vi "getParametresEssai.vi"(8 "error in (no error)":errorcluster, 11 "VISA resource name":refnum<visa-resource-name>) -> (0 "error out":errorcluster, 2 "param out":T1, 3 "VISA resource name out":refnum<visa-resource-name>)   [LabVIEW 2023]
panel:
  out "read buffer":string
  out "Distance (mm)":dbl
  out "vitesse (mm/s)":dbl
  out "temps attente (ms)":i32
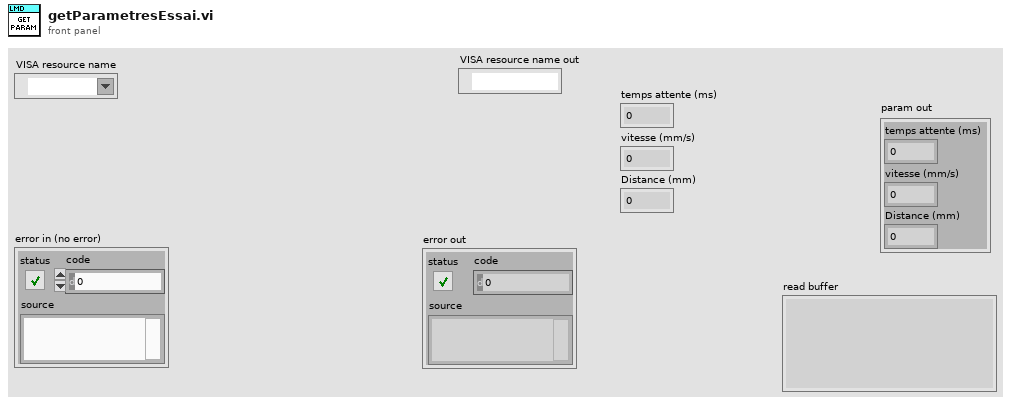
[diagram p1: front panel]
types:
  T1 = cluster{"temps attente (ms)":i32, "vitesse (mm/s)":dbl, "Distance (mm)":dbl}
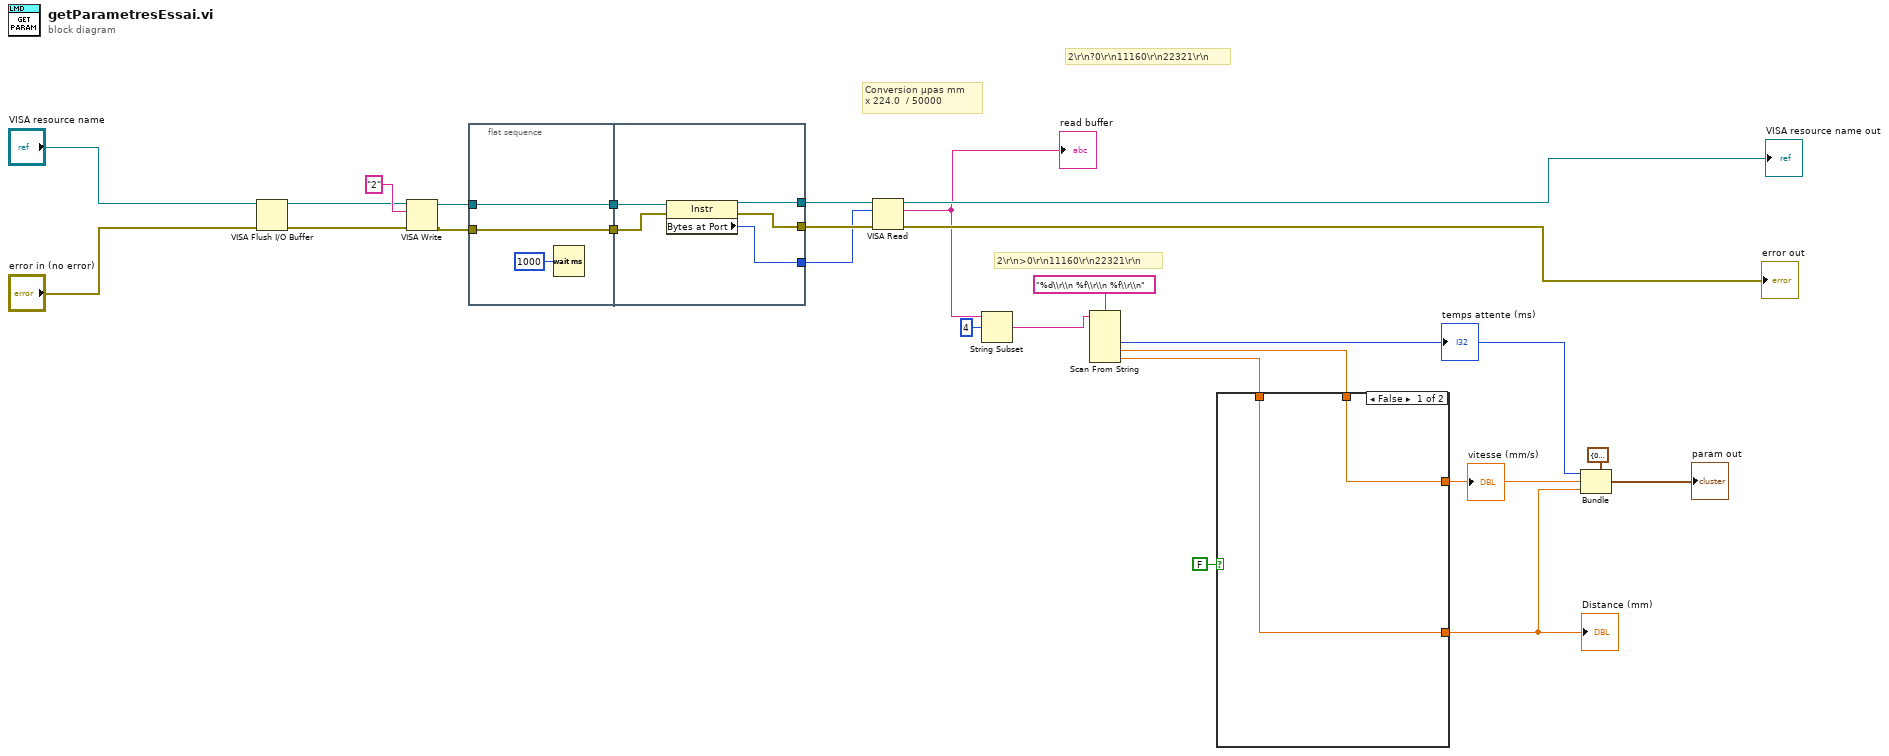
[diagram p0: block diagram]
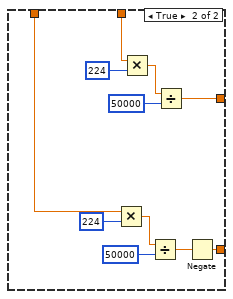
[diagram p2: hidden frame]
diagram:
  # "2\\r\\n>0\\r\\n11160\\r\\n22321\\r\\n"
  # "2\\r\\n?0\\r\\n11160\\r\\n22321\\r\\n"
  # "Conversion µpas mm \nx 224.0  / 50000"
  n1 = VISA Flush I/O Buffer(VISA resource name="VISA resource name", error in (no error)="error in (no error)") -> (VISA resource name out=w3:refnum<visa-resource-name>, error out=w4:errorcluster)  [unwired: 1 in]
  n2 = VISA Write(VISA resource name=w3, write buffer="2", error in (no error)=w4) -> (VISA resource name out=w16:refnum<visa-resource-name>, error out=w13:errorcluster)  [unwired: 1 out]
  n3 = flat-sequence {
    tunnel: w16 -> [w28]
    tunnel: [w28] -> w15
    tunnel: [w27] -> w14
    tunnel: w13 -> [w27]
    tunnel: w15 -> [w34]
    tunnel: w14 -> [w33]
    tunnel: [w32] -> w12
    tunnel: [w31] -> w11
    tunnel: [w30] -> w10
    frame #0 {
      n4 = Wait (ms)(milliseconds to wait=u32 1000) -> ()  [unwired: 1 out]
    }
    frame #1 {
      n5 = property class="Instr"(reference=w34, error in=w33) -> (reference out=w31:refnum<visa-resource-name>, error out=w32:errorcluster, "Bytes at Port"=w30:u32)
    }
  }
  n6 = VISA Read(VISA resource name=w11, byte count=w10, error in (no error)=w12) -> (VISA resource name out=→"VISA resource name out":refnum<visa-resource-name>, read buffer=w9:string, error out=→"error out":errorcluster)  [unwired: 1 out]
  "read buffer" <- w9
  n7 = String Subset(string=w9, offset (0)=4) -> (substring=w7:string)  [unwired: 1 in]
  n8 = Scan From String(format string="%d\\r\\n %f\\r\\n %f\\r\\n", input string=w7) -> (output 1=w19:i32, output 2=w22:dbl, output 3=w21:dbl)  [unwired: 5 in, 3 out]
  "temps attente (ms)" <- w19
  n9 = case shown="False" FALSE {
    tunnel: w22 -> [w36 w41]
    tunnel: w21 -> [w35 w40]
    tunnel: [w36 w39] -> w18
    tunnel: [w35 w37] -> w2
    frame False {
    }
    frame True {
      n10 = Multiply(x=w40, y=224) -> (x*y=w43:dbl)
      n11 = Multiply(x=w41, y=224) -> (x*y=w46:dbl)
      n12 = Divide(x=w43, y=50000) -> (x/y=w38:dbl)
      n13 = Divide(x=w46, y=50000) -> (x/y=w39:dbl)
      n14 = Negate(x=w38) -> (-x=w37:dbl)
    }
  }
  "vitesse (mm/s)" <- w18
  "Distance (mm)" <- w2
  n15 = Bundle(cluster=T1 {"temps attente (ms)"=0, "vitesse (mm/s)"=0.0, "Distance (mm)"=0.0} ("param out"), "temps attente (ms)"=w19, "vitesse (mm/s)"=w18, "Distance (mm)"=w2) -> (→"param out":T1)
